vi "Read CSV File.vi"(3 "error in":errorcluster, 4 "COMSOL CSV File":path=path "C:/Users/plane/Desktop/COMSOL/Data/AllSignals_U_5_5_1e3.csv") -> (0 "error out":errorcluster, 1 "Array":dbl[][](array[numeric]))   [LabVIEW 2013]
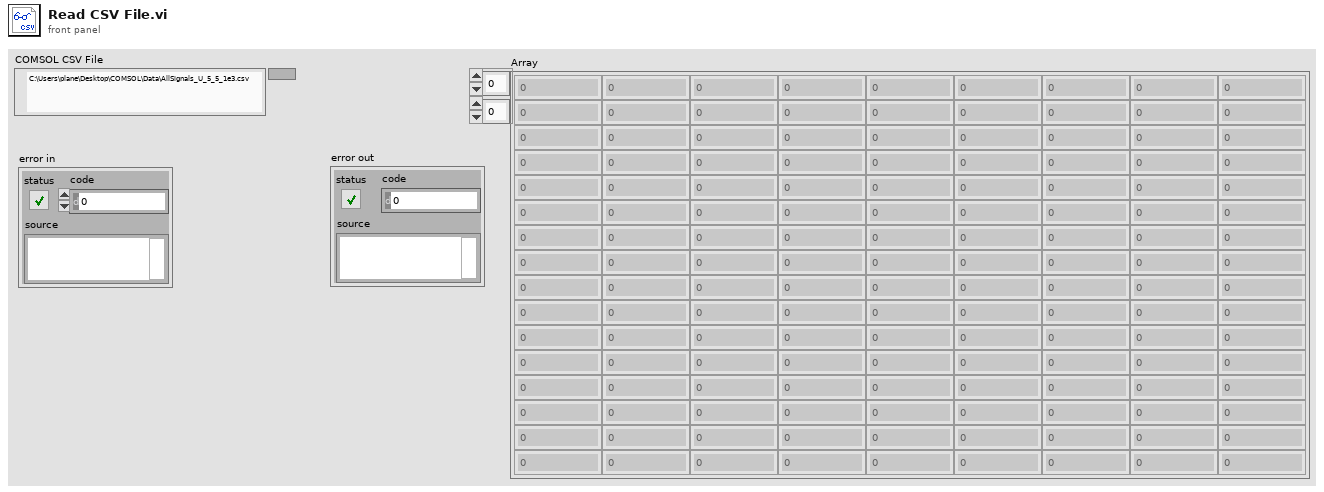
[diagram p1: front panel]
types:
  T1 = enum16{"open", "replace", "create", "open or create", "replace or create", "replace or create with confirmation"}
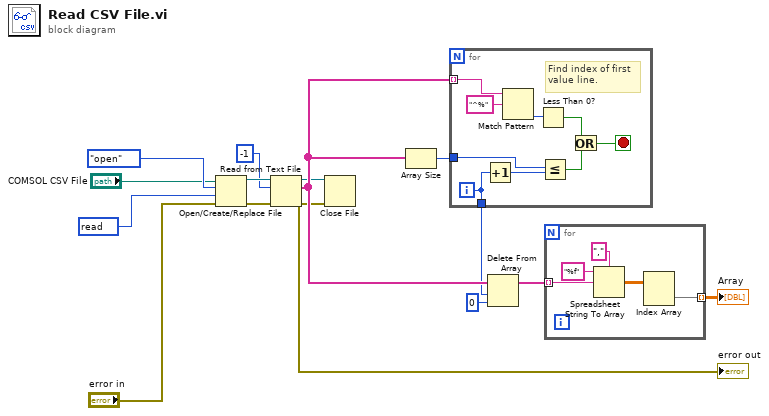
[diagram p0: block diagram]
diagram:
  w15 = u32 2147483648 items=["read"=2147483648, "write"=1073741824, "read & write"=3221225472, "execute"=536870912, "all"=268435456] ("desired access (read & write)")
  n1 = Open/Create/Replace File(file path (use dialog)="COMSOL CSV File", error in="error in", operation (0:open)=T1."open", access (0:read/write)=w15) -> (refnum out=w11:refnum<file>, error out=w10:errorcluster)  [unwired: 2 in, 1 out]
  n2 = Read from Text File(file (use dialog)=w11, count=-1, error in=w10) -> (refnum out=w2:refnum<file>, text=w7:string[], error out=w1:errorcluster)  [unwired: 1 in, 1 out]
  "error out" <- w1
  n3 = Close File(refnum=w2, error in=w1) -> ()  [unwired: 2 out]
  n4 = Array Size(array=w7) -> (size(s)=w8:i32)
  n5 = for {
    tunnel: w7 -> [w22] mode=indexing
    tunnel: w8 -> [w20]
    tunnel: [w17] -> w5
    i -> [w17]
    stop <- w16 stop-if-true
    # "Find index of first\nvalue line."
    n6 = Increment(x=w17) -> (x+1=w21:i32)
    n7 = Match Pattern(string=w22, regular expression="^%") -> (offset past match=w23:i32)  [unwired: 1 in, 3 out]
    n8 = Less Than 0?(x=w23) -> (x < 0?=w18:bool)
    n9 = Less Or Equal?(x=w20, y=w21) -> (x <= y?=w19:bool)
    n10 = Or(x=w18, y=w19) -> (x .or. y?=w16:bool)
  }
  n11 = Delete From Array(array=w7, length=w5, index=0) -> (array with subset deleted=w4:string[])  [unwired: 1 out]
  n12 = for {
    tunnel: w4 -> [w27] mode=indexing
    tunnel: [w25] -> w3 mode=indexing
    n13 = Spreadsheet String To Array(delimiter (Tab)=",", format string="%f", spreadsheet string=w27) -> (array=w26:dbl[][])  [unwired: 1 in]
    n14 = Index Array(array=w26) -> (element=w25:dbl[])  [unwired: 2 in]
  }
  "Array" <- w3
